vi "Elapsed Times.vi"(3 "Call Name":string) -> (1 "Timings":cluster{"Call Name":string, "Delta (ms)":u32}[](array[cluster]))   [LabVIEW 2013]
panel:
  out "GenLog":u32(graph)
  out "Gyro":u32(graph)
  out "Drive":u32(graph)
  out "SM":u32(graph)
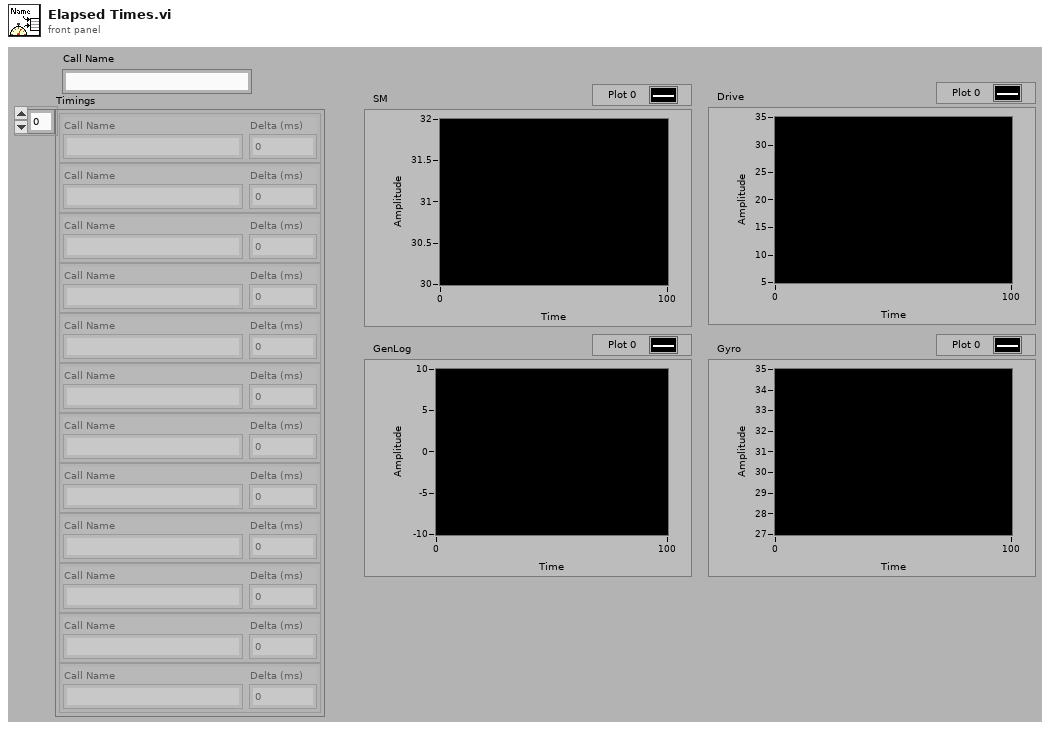
[diagram p1: front panel]
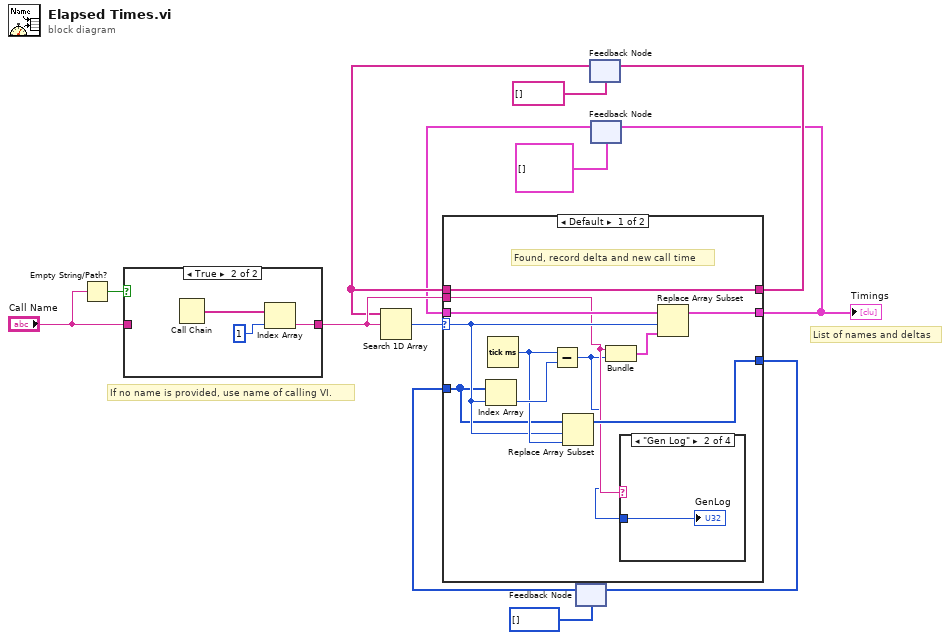
[diagram p0: block diagram]
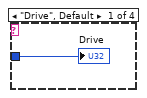
[diagram p2: hidden frame]
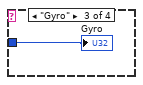
[diagram p3: hidden frame]
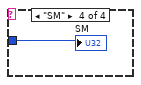
[diagram p4: hidden frame]
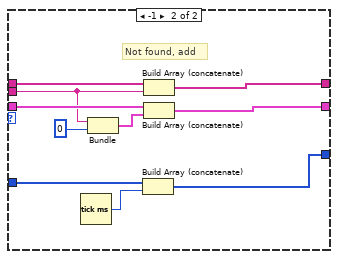
[diagram p5: hidden frame]
diagram:
  # "List of names and deltas"
  # "If no name is provided, use name of calling VI."
  n1 = Empty String/Path?(string/path="Call Name") -> (empty?=w13:bool)
  n2 = case shown="True" w13 {
    tunnel: "Call Name" -> [w14 _]
    tunnel: [w14 w17] -> w10
    frame False {
    }
    frame True {
      n3 = Call Chain() -> (call chain=w16:string[])
      n4 = Index Array(array=w16, index=1 ("millisecond timer value")) -> (element=w17:string)
    }
  }
  n5 = feedback #1(u32[] []) -> (w5:u32[])
  n6 = feedback #2(string[] []) -> (w8:string[])
  n7 = Search 1D Array(1D array=w8, element=w10) -> (index of element=w11:i32)  [unwired: 1 out]
  n8 = feedback #3(cluster{"Name":string, u32}[] []) -> (w2:cluster{"Call Name":string, u32}[])
  n9 = case shown="Default" w11 {
    selector: w11 -> [w22 _]
    tunnel: w10 -> [w19 w35]
    tunnel: [w26 w41] -> w9
    tunnel: w8 -> [w26 w40]
    tunnel: [w20 w39] -> w6
    tunnel: w5 -> [w21 w38]
    tunnel: [w25 w33] -> w3
    tunnel: w2 -> [w24 w37]
    frame Default {
      # "Found, record delta and new call time"
      n10 = Index Array(array=w21, index=w22) -> (element=w28:u32)
      n11 = Tick Count (ms)() -> (millisecond timer value=w23:u32)
      n12 = Subtract(x=w23, y=w28) -> (x-y=w18:u32)
      n13 = Replace Array Subset(array=w21, new element=w23, index=w22) -> (w20:u32[])
      n14 = Bundle("Call Name"=w19, w18) -> (w27:cluster{"Call Name":string, u32})  [unwired: 1 out]
      n15 = case shown="\"Gen Log\"" w19 {
        tunnel: w18 -> [w29 w30 w31 w32]
        frame "Drive", Default {
          "Drive" <- w29
        }
        frame "Gen Log" {
          "GenLog" <- w30
        }
        frame "Gyro" {
          "Gyro" <- w31
        }
        frame "SM" {
          "SM" <- w32
        }
      }
      n16 = Replace Array Subset(array=w24, new element=w27, index=w22) -> (w25:cluster{"Call Name":string, u32}[])
    }
    frame -1 {
      # "Not found, add"
      n17 = Tick Count (ms)() -> (millisecond timer value=w42:u32)
      n18 = Bundle("Call Name"=w35, 0) -> (w34:cluster{"Call Name":string, i32})  [unwired: 1 out]
      n19 = Build Array (concatenate)(w38, w42) -> (w39:u32[])
      n20 = Build Array (concatenate)(w40, w35) -> (w41:string[])
      n21 = Build Array (concatenate)(w37, w34) -> (w33:cluster{"Call Name":string, u32}[])
    }
  }
  "Timings" <- w3
  n22 = feedback-in #1(w6) -> ()
  n23 = feedback-in #2(w9) -> ()
  n24 = feedback-in #3(w3) -> ()
